vi "stop.vi"(8 "error in (no error)":errorcluster, 11 "ClockDL100201DAQmx in":refnum<class "ClockDL100201DAQmx.lvclass">) -> (0 "error out":errorcluster, 3 "ClockDL100201DAQmx out":refnum<class "ClockDL100201DAQmx.lvclass">)   [LabVIEW 2010, in "ClockDL100201DAQmx.lvclass"]
uses:
  ClockDL100201DAQmx.lvclass
  ClockDL100201DAQmx.lvclass/ClockDL100201DAQmx.ctl
  GenericClock/GenericClock/GenericClock.lvclass
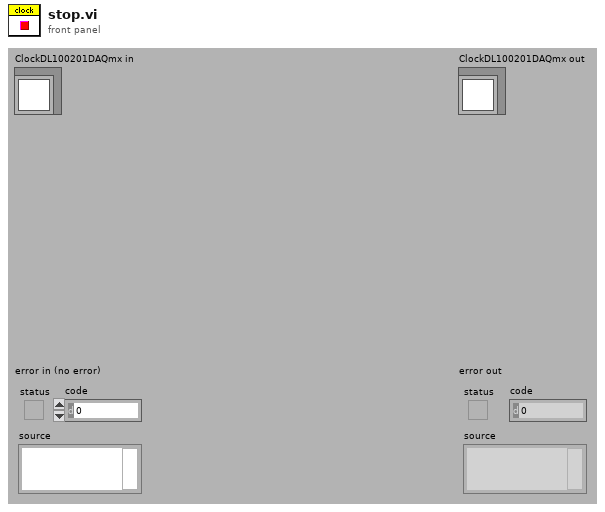
[diagram p1: front panel]
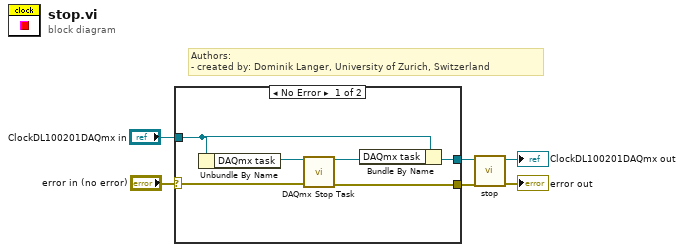
[diagram p0: block diagram]
diagram:
  # "Authors: \n- created by: Dominik Langer, University of Zurich, Switzerland"
  n1 = case shown="No Error" "error in (no error)" {
    selector: "error in (no error)" -> [w12 w13]
    tunnel: [w11 w13] -> w3
    tunnel: "ClockDL100201DAQmx in" -> [w9 w14]
    tunnel: [w7 w14] -> w1
    frame No Error {
      n2 = Unbundle By Name(w9) -> ("DAQmx task"=w10:refnum<k21>)
      n3 = call <vilib>:"DAQmx Stop Task.vi"("task/channels in"=w10, "error in"=w12) -> ("task out"=w8:refnum<k21>, "error out"=w11:errorcluster)  [unwired: 12 in]
      n4 = Bundle By Name(cluster=w9, "DAQmx task"=w8) -> (w7:refnum<class "ClockDL100201DAQmx.lvclass">)
    }
    frame Error {
    }
  }
  n5 = call-parent "stop.vi"("error in (no error)"=w3, "GenericClock in"=w1) -> ("error out"=→"error out":errorcluster, "GenericClock out"=→"ClockDL100201DAQmx out":refnum<class "ClockDL100201DAQmx.lvclass">)  [unwired: 8 in]
